vi "write single relay.vi"(8 "error in (no error)":errorcluster, 9 "High/Low":bool, 10 "Line Enum":T1, 11 "USB IO in":refnum<class "USB IO.lvclass">) -> (0 "error out":errorcluster, 3 "USB IO out":refnum<class "USB IO.lvclass">)   [LabVIEW 2025, in "USB IO.lvclass"]
uses:
  USB IO.lvclass
  USB IO.lvclass/USB IO.ctl
  dqmh-lvoop-template/Classes/Data Log/Line.ctl
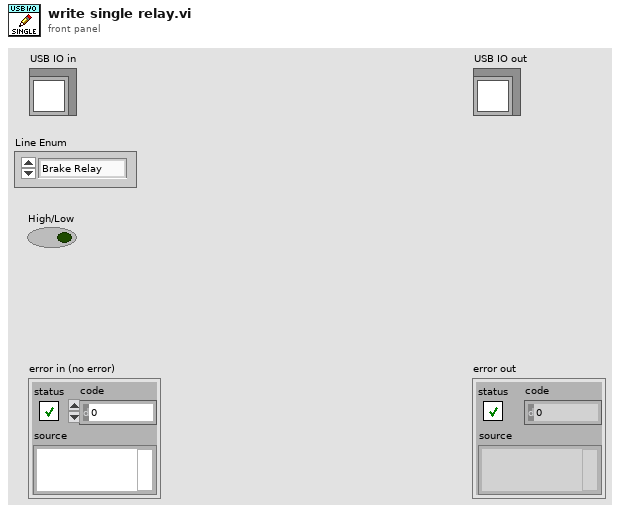
[diagram p1: front panel]
types:
  T1 = typedef "USB IO.lvclass/Line.ctl" = enum16{"Brake Relay", "PS Relay"}
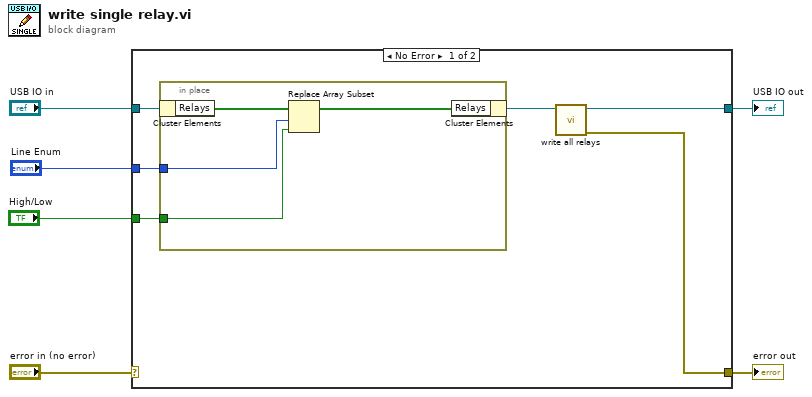
[diagram p0: block diagram]
diagram:
  n1 = case shown="No Error" "error in (no error)" {
    selector: "error in (no error)" -> [_ w18]
    tunnel: [w7 w18] -> w5
    tunnel: [w8 w17] -> w3
    tunnel: "USB IO in" -> [w12 w17]
    tunnel: "Line Enum" -> [w11 _]
    tunnel: "High/Low" -> [w10 _]
    frame No Error {
      n2 = in-place {
        in-place-border: w11 -> [w15]
        in-place-border: w10 -> [w14]
        n3 = in-place-cluster #1(w12) -> ("Relays"=w16:bool[])
        n4 = Replace Array Subset(array=w16, new element=w14, index=w15) -> (w13:bool[])
        n5 = in-place-cluster #1("Relays"=w13) -> (w9:refnum<class "USB IO.lvclass">)
      }
      n6 = call-dynamic "write all relays.vi"("USB IO in"=w9) -> ("error out"=w7:errorcluster, "USB IO out"=w8:refnum<class "USB IO.lvclass">)  [unwired: 9 in]
    }
    frame Error {
    }
  }
  "error out" <- w5
  "USB IO out" <- w3
